vi "SeCrTs-AI_V_Read.vi"(7 "Data FIFO Ref":T1, 8 "error in":errorcluster, 10 "number of samples per channel":i32=51, 11 "AI_V_Task":refnum<k21>) -> (0 "error out":errorcluster, 3 "AI_V_Task":refnum<k21>)   [LabVIEW 2022 SP3]
uses:
  RT Controls/ATF Storage-Data FIFO.ctl
  RT Controls/ATF Storage Haelth.ctl
  <vilib>/DAQmx/read.llb/DAQmx Read (Analog 1D Wfm NChan NSamp).vi
  <vilib>/DAQmx/miscellaneous.llb/DAQmx Fill In Error Info.vi
panel:
  out "overflow?":bool
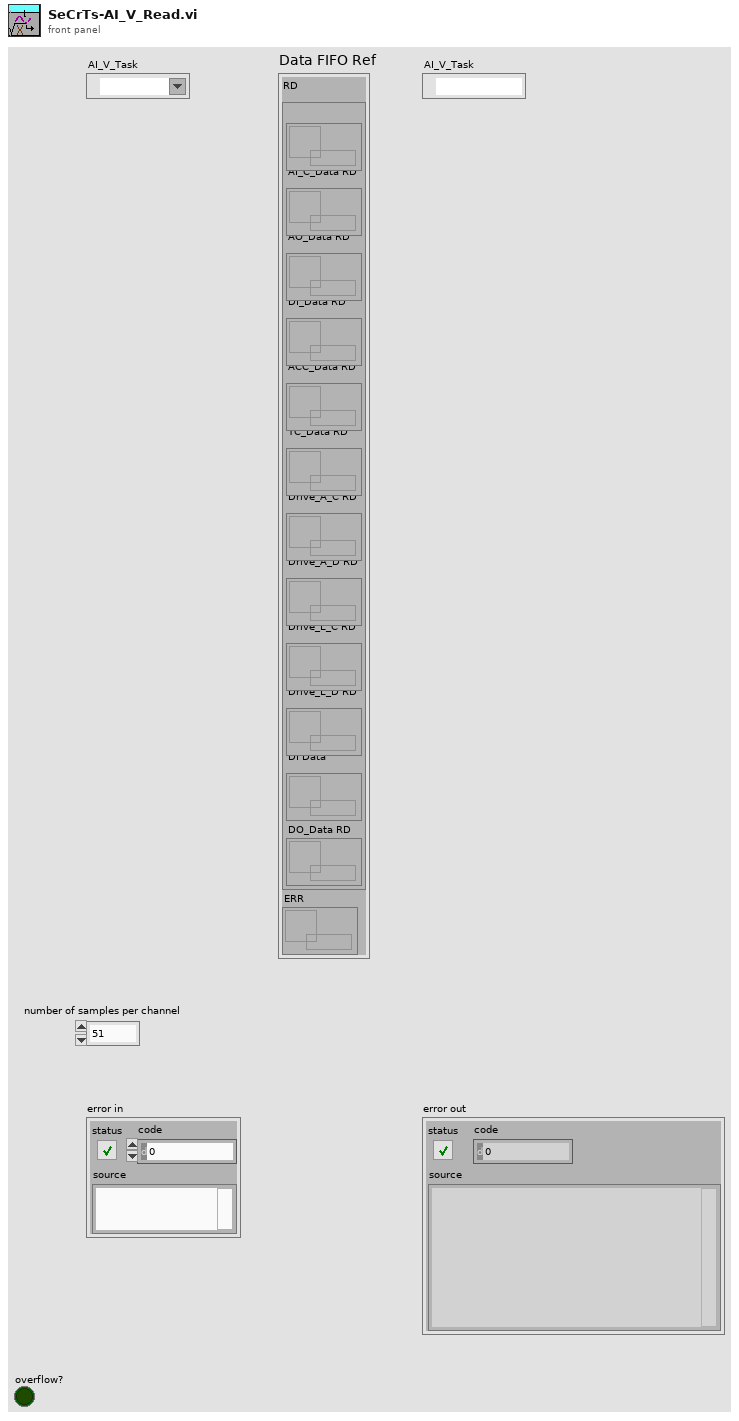
[diagram p1: front panel]
types:
  T1 = typedef "ATF Storage-Data FIFO.ctl" = cluster{"RD":cluster{"AI_V_Data RD":refnum<queue>, "AI_C_Data RD":refnum<queue>, "AO_Data RD":refnum<queue>, "DI_Data RD":refnum<queue>, "ACC_Data RD":refnum<queue>, "TC_Data RD":refnum<queue>, "Drive_A_C RD":refnum<queue>, "Drive_A_D RD":refnum<queue>, "Drive_L_C RD":refnum<queue>, "Drive_L_D RD":refnum<queue>, "DI Data":refnum<queue>, "DO_Data RD":refnum<queue>}, "ERR":refnum<queue>}
  T2 = cluster{"AO config":cluster{"Channel_Name":string, "Channel_Number":string, "Default_Value":dbl, "Units":string}[], "AI config":cluster{"Channel_Name":string, "Channel_Number":string, "Pre_Scale_min":dbl, "Pre_Scale_max":dbl, "Sensor_min":dbl, "Sensor_max":dbl, "Units":string}[], "DI config":cluster{"Channel_Name":string, "Channel_Number":string, "Default_Value":bool, "DI invert?":bool}[], "DO config":cluster{"Channel_Name":string, "Channel_Number":string, "Default_Value":bool, "DO invert?":bool}[], "TC config":cluster{"Channel_Name":string, "Channel_Number":string, "Pre_Scale_min":dbl, "Pre_Scale_max":dbl, "units":i32, "thermocouple type":i32}[], "ACC config":cluster{"Channel_Name":string, "Channel_Number":string, "Pre_Scale_min":dbl, "Pre_Scale_max":dbl, "Terminal configuration":i32, "Sensitivity":dbl, "Sensitivity units":i32}[], "SG config":cluster{"Channel_Name":string, "Channel_Number":string, "Pre_Scale_min":dbl, "Pre_Scale_max":dbl}[], "Strain Gauge Settings":cluster{"poisson ratio":dbl, "nominal gage resistance":dbl, "gage factor":dbl}, "Bridge Settings":cluster{"voltage excitation value":dbl, "voltage excitation source":i32, "initial bridge voltage":dbl, "lead wire resistance":dbl, "strain configuration":i32}, "Sample Rate":cluster{"AI Sample Rate":dbl[], "AO Sample Rate":dbl[], "DI Sample Rate":dbl[], "TC Sample Rate":dbl[], "DO Sample Rate":dbl[], "SG Sample Rate":dbl[], "ACC Sample Rate":dbl[]}}
  T3 = cluster{"Channel_Name":string, "Channel_Number":string, "Pre_Scale_min":dbl, "Pre_Scale_max":dbl, "Sensor_min":dbl, "Sensor_max":dbl, "Units":string}[]
  T4 = typedef "ATF Storage Haelth.ctl" = enum16{"AI C", "AI V", "AO", "DI", "DO", "TC", "ACC", "RT Str", "DR A"}
  T5 = enum16{"Init", "Read 'All'", "Read 'n'", "Read '1'", "Write '1'", "Write 'n'", "Write 'All'"}
  T6 = cluster{"Start DAQ":bool, "Stop DAQ":bool, "RT Stop":bool, "RT Exit":bool, "Start Seq":bool}
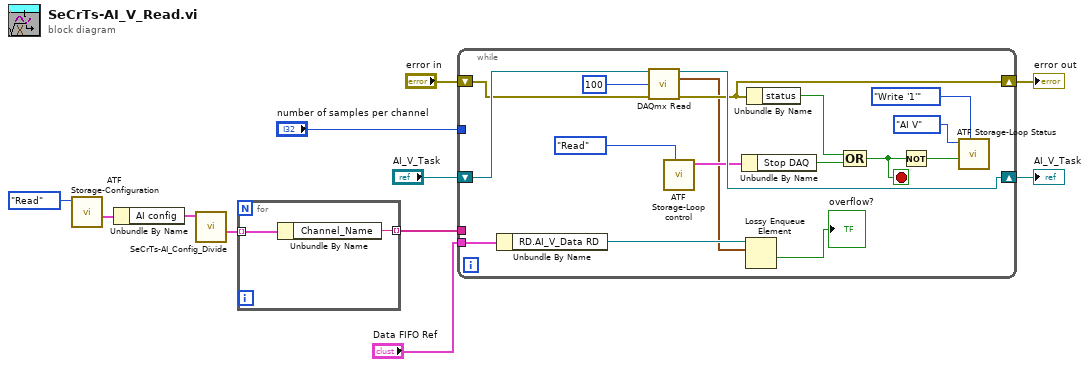
[diagram p0: block diagram]
diagram:
  n1 = call "ATF Storage-Configuration.vi"("Enum"=enum16{"Write", "Read"}."Read") -> ("Config out"=w4:T2)  [unwired: 10 in]
  n2 = Unbundle By Name(w4) -> ("AI config"=w3:T3)
  n3 = call "SeCrTs-AI_Config_Divide.vi"("AI config"=w3) -> ("AI C"=w2:T3)  [unwired: 9 in, 1 out]
  n4 = for {
    tunnel: w2 -> [w13] mode=indexing
    tunnel: [w12] -> w1 mode=indexing
    n5 = Unbundle By Name(w13) -> ("Channel_Name"=w12:string)
  }
  n6 = while {
    shift-right: [w28] -> w6
    shift-left: "AI_V_Task" -> [w30]
    shift-right: [w27] -> w9
    shift-left: "error in" -> [w29]
    tunnel: "number of samples per channel" -> [_]
    tunnel: "Data FIFO Ref" -> [w21]
    tunnel: w1 -> [_]
    stop <- w26 stop-if-true
    n7 = Unbundle By Name(w21) -> ("RD.AI_V_Data RD"=w18:refnum<queue>)
    n8 = call-poly <vilib>:"DAQmx Read.vi"("task/channels in"=w30, "number of samples per channel"=100, "error in"=w29) -> ("task out"=w28:refnum<k21>, "data"=w15:waveform(dbl)[], "error out"=w27:errorcluster)  [unwired: 10 in]
    n9 = call "ATF Storage-Loop control.vi"("Action"=enum16{"Init", "Write", "Read"}."Read") -> ("Loop Control out"=w24:T6)  [unwired: 9 in, 1 out]
    n10 = Unbundle By Name(w24) -> ("Stop DAQ"=w23:bool)
    n11 = Lossy Enqueue Element(queue=w18, element=w15) -> (overflow?=→"overflow?":bool)  [unwired: 1 in, 3 out]
    n12 = Unbundle By Name(w27) -> ("status"=w25:bool)
    n13 = Compound Arithmetic op=OR(w25, w23) -> (w26:bool)
    n14 = Not(x=w26) -> (.not. x?=w19:bool)
    n15 = call "ATF Storage-Loop Status.vi"("Option"=T5."Write '1'", "Status"=w19, "Loop"=ATF_Storage_Haelth."AI V") -> ()  [unwired: 6 in, 3 out]
  }
  "error out" <- w9
  "AI_V_Task" <- w6
